vi "Build URI from Components.vi"(8 "error in":errorcluster, 11 "URI Components":T1) -> (0 "error out":errorcluster, 3 "URI":string)   [LabVIEW 2013, in "openURI.lvlib"]
uses:
  openURI.lvlib
  URI Components -- cluster.ctl
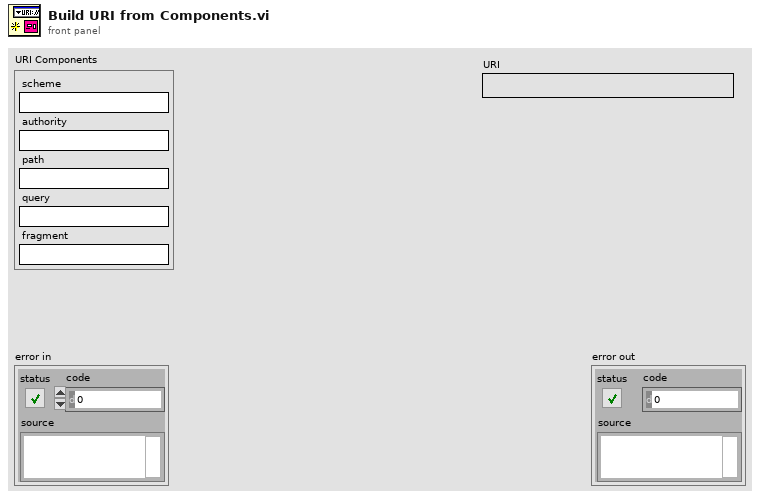
[diagram p1: front panel]
types:
  T1 = typedef "openURI.lvlib/URI Components -- cluster.ctl" = cluster{"scheme":string, "authority":string, "path":string, "query":string, "fragment":string}
  T2 = enum16{"scheme", "authority", "path", "query", "fragment"}
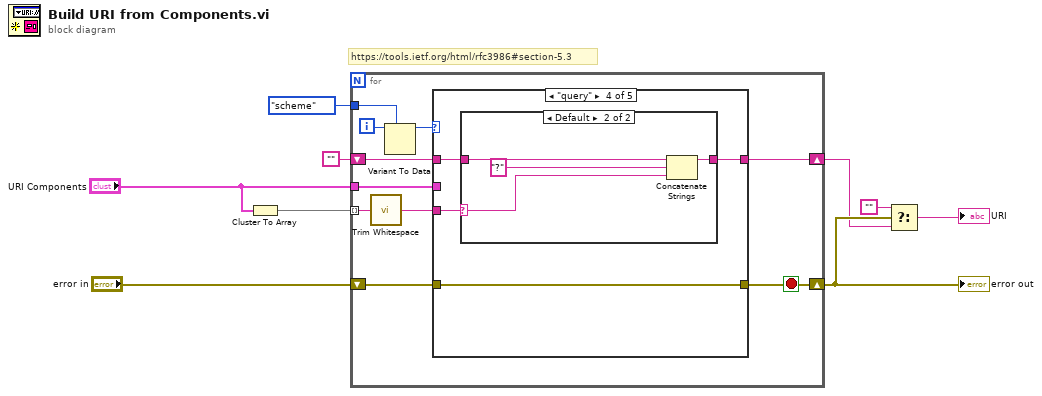
[diagram p0: block diagram]
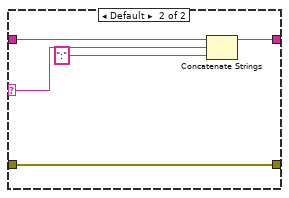
[diagram p3: hidden frame]
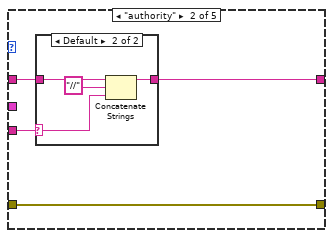
[diagram p4: hidden frame]
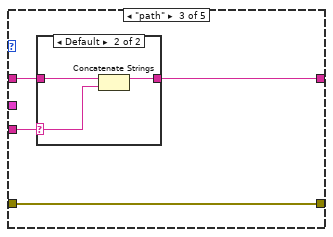
[diagram p6: hidden frame]
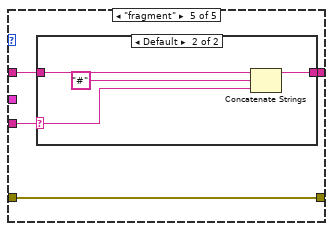
[diagram p9: hidden frame]
diagram:
  # "https://tools.ietf.org/html/rfc3986#section-5.3"
  n1 = Cluster To Array(cluster="URI Components") -> (array=w7:string[])
  n2 = for {
    tunnel: w7 -> [w17] mode=indexing
    shift-right: [w16] -> w4
    shift-left: "" -> [w18]
    tunnel: T2."scheme" -> [w14]
    tunnel: "URI Components" -> [w12]
    shift-right: [w10] -> w5
    shift-left: "error in" -> [w11]
    i -> [w15]
    stop <- w10 stop-if-true
    n3 = call <vilib>:"Trim Whitespace.vi"("string"=w17) -> ("trimmed string"=w19:string)  [unwired: 1 in]
    n4 = Variant To Data(type=w14, Variant=w15) -> (data=w13:T2)  [unwired: 1 in, 1 out]
    n5 = case shown="\"query\"" w13 {
      tunnel: w19 -> [w24 w35 w44 w52 w61]
      tunnel: w18 -> [w23 w34 w43 w51 w60]
      tunnel: [w22 w33 w42 w50 w59] -> w16
      tunnel: w12 -> [_ _ _ _ _]
      tunnel: [w21 w32 w41 w49 w58] -> w10
      tunnel: w11 -> [w20 w32 w41 w49 w58]
      frame "scheme" {
        n6 = case shown="\"\"" w24 {
          selector: w24 -> [_ w30]
          tunnel: w23 -> [w26 w31]
          tunnel: [w26 w28] -> w22
          tunnel: [w25 w27] -> w21
          tunnel: w20 -> [w25 w27]
          frame "" {
            # "#TODO: \nhttps://tools.ietf.org/html/rfc3986#section-3"
          }
          frame Default {
            n7 = Concatenate Strings(w31, w30, ":" ("string")) -> (w28:string)
          }
        }
      }
      frame "authority" {
        n8 = case shown="Default" w35 {
          selector: w35 -> [_ w37]
          tunnel: w34 -> [w36 w40]
          tunnel: [w36 w39] -> w33
          frame "" {
          }
          frame Default {
            n9 = Concatenate Strings(w40, "//" ("string"), w37) -> (w39:string)
          }
        }
      }
      frame "path" {
        n10 = case shown="Default" w44 {
          selector: w44 -> [_ w46]
          tunnel: w43 -> [w45 w48]
          tunnel: [w45 w47] -> w42
          frame "" {
          }
          frame Default {
            n11 = Concatenate Strings(w48, w46) -> (w47:string)
          }
        }
      }
      frame "query" {
        n12 = case shown="Default" w52 {
          selector: w52 -> [_ w54]
          tunnel: w51 -> [w53 w57]
          tunnel: [w53 w56] -> w50
          frame "" {
          }
          frame Default {
            n13 = Concatenate Strings(w57, "?" ("string"), w54) -> (w56:string)
          }
        }
      }
      frame "fragment" {
        n14 = case shown="Default" w61 {
          selector: w61 -> [_ w63]
          tunnel: w60 -> [w62 w66]
          tunnel: [w62 w65] -> w59
          frame "" {
          }
          frame Default {
            n15 = Concatenate Strings(w66, "#" ("string"), w63) -> (w65:string)
          }
        }
      }
    }
  }
  "error out" <- w5
  n16 = Select(t="", s=w5, f=w4) -> (s? t:f=→"URI":string)
